vi "rethinkdb_json_has_keys.vi"(10 "keys to find":string[](array[string]), 11 "json":string) -> (3 "keys found?":bool)   [LabVIEW 2017]
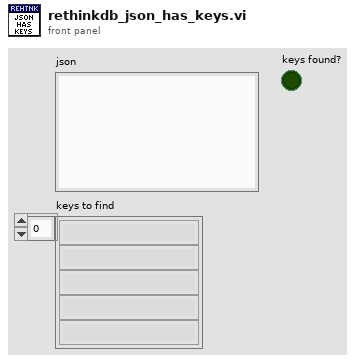
[diagram p1: front panel]
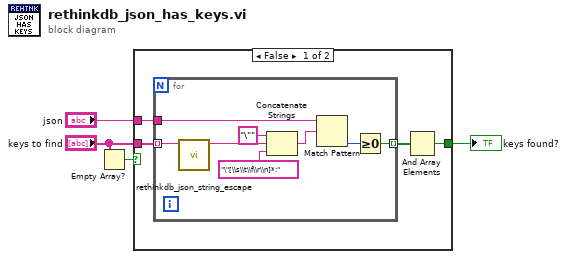
[diagram p0: block diagram]
diagram:
  n1 = Empty Array?(array="keys to find") -> (empty?=w1:bool)
  n2 = case shown="False" w1 {
    tunnel: "json" -> [w8 _]
    tunnel: "keys to find" -> [w7 _]
    tunnel: [w5 _] -> w3
    frame False {
      n3 = for {
        tunnel: w8 -> [w16]
        tunnel: w7 -> [w15] mode=indexing
        tunnel: [w9] -> w6 mode=indexing
        n4 = call "rethinkdb_json_string_escape.vi"("string"=w15) -> ("escaped string"=w14:string)  [unwired: 10 in]
        n5 = Concatenate Strings("\"" ("string"), w14, "\"[\\s\\t\\f\\r\\n]*:" ("string")) -> (w11:string)
        n6 = Match Pattern(string=w16, regular expression=w11) -> (offset past match=w10:i32)  [unwired: 1 in, 3 out]
        n7 = Greater Or Equal To 0?(x=w10) -> (x >= 0?=w9:bool)
      }
      n8 = And Array Elements(Boolean array=w6) -> (logical AND=w5:bool)
    }
    frame True {
    }
  }
  "keys found?" <- w3
